vi "Test_WriteValue_CheckItemNames_NamesUpdated.vi"(8 "error in (no error)":errorcluster, 11 "TestCase in":refnum<class "TestListboxItemNamesBinding.lvclass">) -> (0 "error out":errorcluster, 3 "TestCase out":refnum<class "TestListboxItemNamesBinding.lvclass">)   [LabVIEW 2017, in "TestListboxItemNamesBinding.lvclass"]
uses:
  TestListboxItemNamesBinding.lvclass
  Source/Concrete/ListboxItemNamesBinding/ListboxItemNamesBinding.lvclass/ListboxItemNamesBinding.ctl
  Source/Concrete/ListboxItemNamesBinding/ListboxItemNamesBinding.lvclass
  C:/Git/composed-transport/Source/ITransport/ITransport.lvclass
  <vilib>/Utility/error.llb/Error Cluster From Error Code.vi
  Source/ITransport/ITransport.lvclass
panel:
  in  "Listbox":i32(listbox)
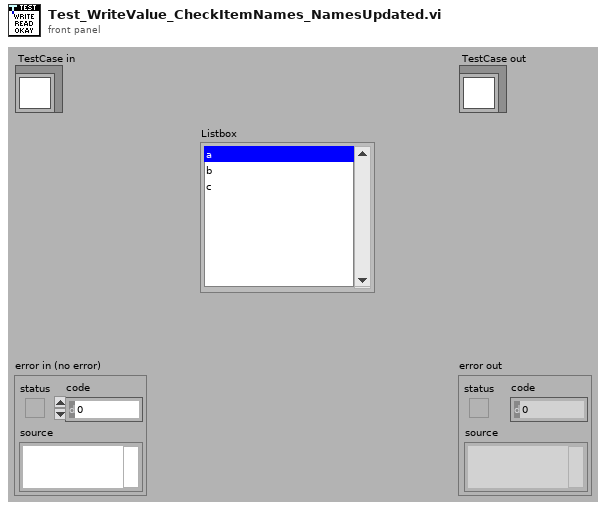
[diagram p1: front panel]
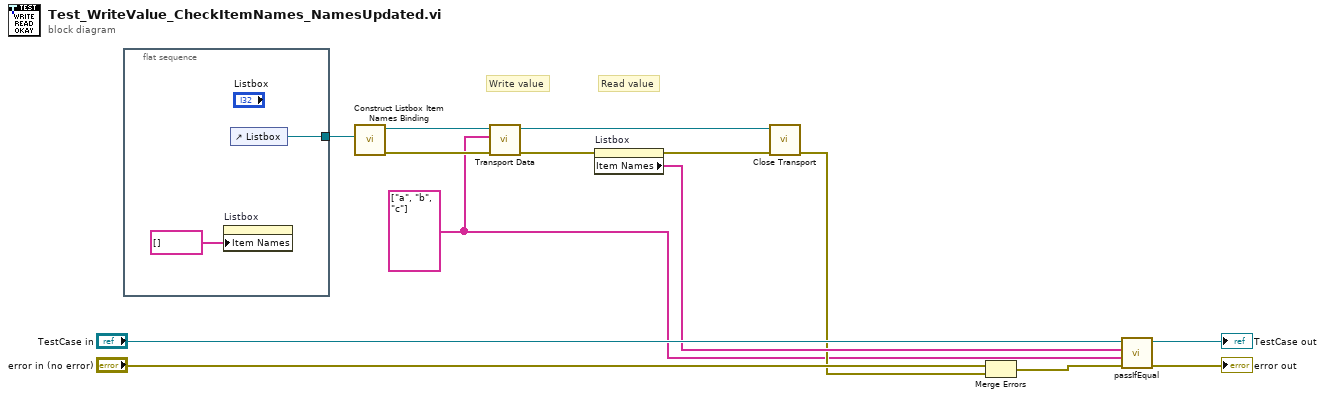
[diagram p0: block diagram]
diagram:
  w1 = string[] ["a", "b", "c"]
  # "Read value"
  # "Write value"
  n1 = flat-sequence {
    tunnel: [w16] -> w6
    frame #0 {
      n2 = property on="Listbox" class="LstBox (strict)"("Item Names"=string[] []) -> ()  [unwired: 2 in, 2 out]
      n3 = control-ref of="Listbox"() -> (w16:refnum<vi>)
    }
  }
  n4 = call "Construct Listbox Item Names Binding.vi"("LstBox Refnum"=w6) -> ("error out"=w8:errorcluster, "ListboxItemNamesBinding"=w10:refnum<class "ListboxItemNamesBinding.lvclass">)  [unwired: 9 in]
  n5 = call "Transport Data.vi"("error in (no error)"=w8, "Value"=w1, "ITransport in"=w10) -> ("error out"=w5:errorcluster, "ITransport out"=w7:refnum<class "ListboxItemNamesBinding.lvclass">)  [unwired: 7 in]
  n6 = property on="Listbox" class="LstBox (strict)"(error in=w5) -> (error out=w4:errorcluster, "Item Names"=w3:string[])  [unwired: 1 in, 1 out]
  n7 = call-dynamic "Close Transport.vi"("error in (no error)"=w4, "ITransport in"=w7) -> ("error out"=w2:errorcluster)  [unwired: 9 in]
  n8 = Merge Errors("error in (no error)", w2) -> (w9:errorcluster)
  n9 = call-dynamic "passIfEqual.vi"("error in (no error)"=w9, "y"=w1, "x"=w3, "TestCase in"="TestCase in") -> ("error out"=→"error out":errorcluster, "TestCase out"=→"TestCase out":refnum<class "TestListboxItemNamesBinding.lvclass">)  [unwired: 6 in]
